vi "Video Write.vi"() -> ()   [LabVIEW 2020, in "examples.lvlib"]
uses:
  examples.lvlib
  common/Image Size (Integer).ctl
  video_io/FourCC.ctl
  video_io/Writer (ARGB)/Writer (ARGB).lvclass/Writer (ARGB).ctl
  common/Image Point (Integer).ctl
  image/Text Drawing Settings.ctl
  image/Font Face.ctl
  image/ARGB Colour.ctl
  video_io/Reader/Reader.lvclass/Reader.ctl
  image/New Image (ARGB Preallocated).vi
  image/Draw Rectangle (ARGB).vi
  image/Draw Text (ARGB).vi
  image/Draw Image to Picture (ARGB).vi
  video_io/Reader/Read Frame (ARGB Next).vi
  video_io/CreateWriter.vi
  image/New Image (ARGB Preallocated).vi/3321fa97-f432-4e1e-8db9-a0df79aed21b.vi
  image/ARGB Colour to U32 Pixel Value.vi
  image/Draw Rectangle (ARGB).vi/7e6fb015-3761-4366-a0a7-e436eb229083.vi
  image/Draw Text (ARGB).vi/0015c4fc-6a12-4f82-815b-6c2f827f408b.vi
  video_io/Writer (ARGB)/Write Frame.vi/0e3f49b0-4303-46d3-b8ab-944fedc4b55e.vi
  image/Draw Image to Picture (ARGB).vi/8cd07b1b-062e-4fe4-9e87-2eb3dc89fe0e.vi
  video_io/Reader/Read Frame (ARGB Next).vi/9eeb12df-7581-4bcd-a397-18dbd97d2298.vi
  <vilib>/Utility/error.llb/Error Cluster From Error Code.vi
  video_io/Writer (ARGB)/Writer (ARGB).lvclass
  video_io/Reader/Reader.lvclass
  video_io/video_io.lvlib
  image/image.lvlib
  common/common.lvlib
panel:
  out "Size":i64 format="%d kB"
  out "Results":cluster{"Input":picture, "Output":picture}[](array[cluster])
  in  "File and Encoding Option":T1(ring)
  # "Different Containers support different encoding types\n(these are just some examples)"
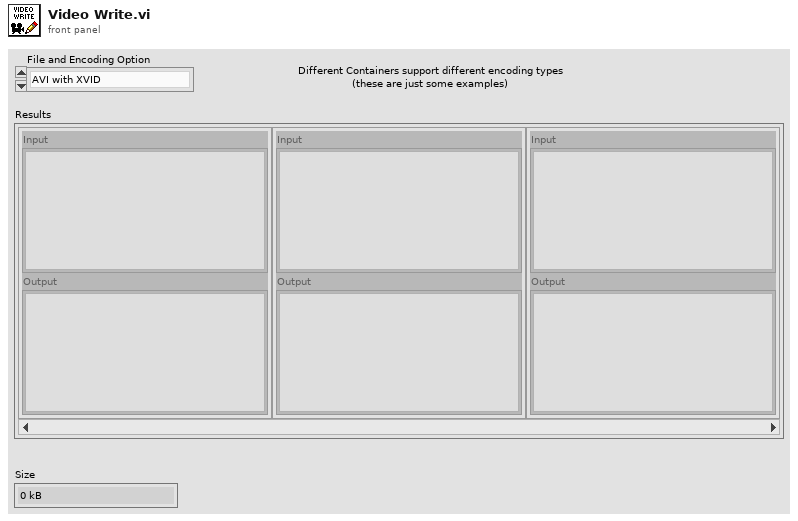
[diagram p1: front panel]
types:
  T1 = enum16{"AVI with XVID", "MKV with RGBA", "MP4 with MP4V"}
  T2 = typedef "common.lvlib/Image Size (Integer).ctl" = cluster{"Width":u16, "Height":u16}
  T3 = typedef "video_io.lvlib/FourCC.ctl" = enum16{"YUV2", "2VUY", "YUVS", "RGBA", "YUV4", "JPEG", "MJPA", "AVDJ", "DMB1", "MP4V", "DIVX", "XVID", "3IV2", "S263", "AVC1", "AI5P", "AI5Q", "AI52", "AI53", "AI55", "AI56", "AI1P", "AI1Q", "AI12", "AI13", "AI15", "AI16", "M1V1", "MPEG", "M2V1", "HDV1", "HDV2", "HDV3", "HDV4", "HDV5", "HDV6", "HDV7", "HDV8", "HDV9", "HDVA", "MX5N", "MX5P", "MX4N", "MX4P", "MX3N", "MX3P", "XD54", "XD55", "XD59", "XD5A", "XD5B", "XD5C", "XD5D", "XD5E", "XD5F", "XDV1", "XDV2", "XDV3", "XDV4", "XDV5", "XDV6", "XDV7", "XDV8", "XDV9", "XDVA", "XDVB", "XDVC", "XDVD", "XDVE", "XDVF", "XDHD", "XDH2", "AVMP", "MJP2", "TIFF", "DRAC", "3IVD", "L555", "L565", "B565", "24BG", "BGRA", "ABGR", "B16G", "B48R", "BXBG", "BXRG", "BXYV", "NO16", "DVOO", "R420", "R411", "WRAW", "AV1X", "AVUP"}
  T4 = typedef "image.lvlib/ARGB Image.ctl" = refnum<data-value>
  T5 = typedef "common.lvlib/Image Point (Integer).ctl" = cluster{"x":i32, "y":i32}
  T6 = typedef "image.lvlib/ARGB Colour.ctl" = cluster{"Alpha":u8, "RGB":u32}
  T7 = typedef "image.lvlib/Text Drawing Settings.ctl" = cluster{"OpenCV Font Face":T8, "Font Scale":dbl}
  T8 = typedef "image.lvlib/Font Face.ctl" = enum8{"FONT_HERSHEY_SIMPLEX", "FONT_HERSHEY_PLAIN", "FONT_HERSHEY_DUPLEX", "FONT_HERSHEY_COMPLEX", "FONT_HERSHEY_TRIPLEX", "FONT_HERSHEY_COMPLEX_SMALL", "FONT_HERSHEY_SCRIPT_SIMPLEX", "FONT_HERSHEY_SCRIPT_COMPLEX", "FONT_ITALIC"}
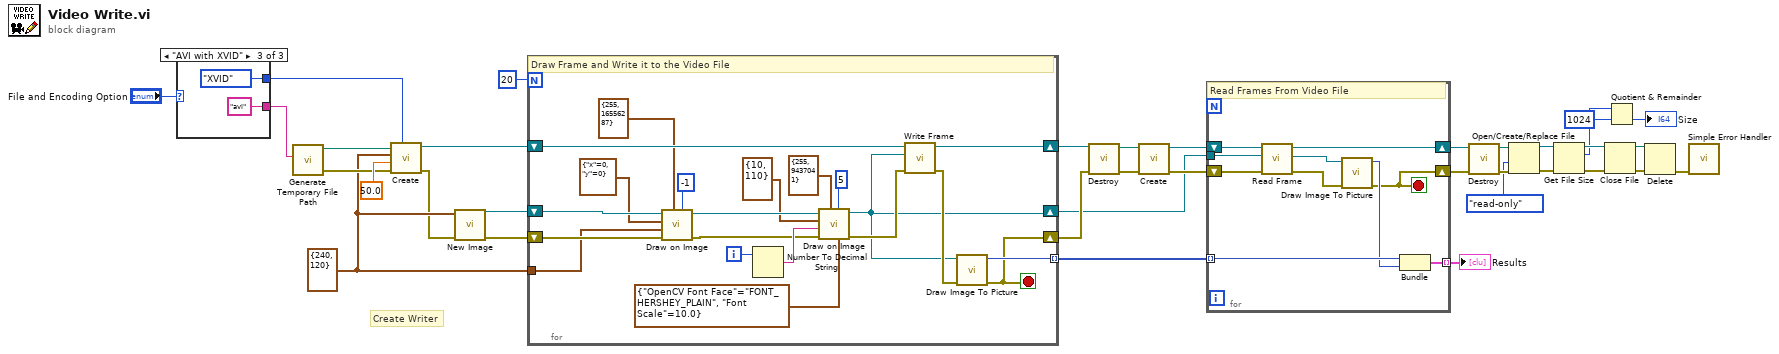
[diagram p0: block diagram]
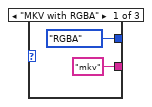
[diagram p2: hidden frame]
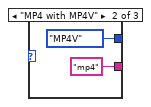
[diagram p3: hidden frame]
diagram:
  w21 = T2 {"Width"=240, "Height"=120} ("Preallocated Image Size (Default: 0,0)")
  # "Create Writer"
  n1 = case shown="\"AVI with XVID\"" "File and Encoding Option" {
    tunnel: ["mkv" "mp4" "avi"] -> w32
    tunnel: [FourCC."RGBA" ("Fourcc") FourCC."MP4V" ("Fourcc") FourCC."XVID" ("Fourcc")] -> w31
    frame "MKV with RGBA" {
    }
    frame "MP4 with MP4V" {
    }
    frame "AVI with XVID" {
    }
  }
  n2 = call <vilib>:"Generate Temporary File Path.vi"("Temporary File Extension (tmp)"=w32) -> ("error out"=w22:errorcluster, "Unique Temporary File Path"=w20:path)  [unwired: 9 in]
  n3 = call "Create.vi"("Fourcc"=w31, "error in (no error)"=w22, "Frames Per Second"=50.0, "Image Size"=w21, "Path"=w20) -> ("error out"=w18:errorcluster, "Writer (ARGB)"=w36:refnum<class "Writer (ARGB).lvclass">)  [unwired: 5 in]
  n4 = call-poly "New Image.vi"("error in (no error)"=w18, "Preallocated Image Size (Default: 0,0)"=w21) -> ("error out"=w17:errorcluster, "ARGB Image"=w27:T4)  [unwired: 8 in]
  n5 = for {
    N: 20 -> [_]
    shift-right: [w53] -> w24
    shift-left: w36 -> [w51]
    shift-right: [w43] -> w34
    shift-left: w17 -> [w55]
    tunnel: w21 -> [w48]
    tunnel: [w45] -> w15 mode=indexing
    shift-right: [w44] -> w16
    shift-left: w27 -> [w61]
    i -> [w57]
    stop <- w43 stop-if-true
    # "Draw Frame and Write it to the Video File"
    n6 = call-poly "Draw on Image.vi"("Thickness (Default: 1)"=-1, "ARGB Colour"=T6 {"Alpha"=255, "RGB"=16556287}, "error in (no error)"=w55, "Point B"=w48, "Point A"=T5 {"x"=0, "y"=0}, "ARGB Image in"=w61) -> ("error out"=w54:errorcluster, "ARGB Image"=w60:T4)  [unwired: 4 in]
    n7 = Number To Decimal String(number=w57) -> (decimal integer string=w56:string)  [unwired: 1 in]
    n8 = call-poly "Draw on Image.vi"("Text Drawing Settings (Default: Simplex)"=T7 {"OpenCV Font Face"=enum."FONT_HERSHEY_PLAIN", "Font Scale"=10.0}, "Thickness (Default: 1)"=5, "ARGB Colour"=T6 {"Alpha"=255, "RGB"=9437041}, "error in (no error)"=w54, "Text"=w56, "Origin"=T5 {"x"=10, "y"=110}, "ARGB Image in"=w60) -> ("error out"=w62:errorcluster, "ARGB Image"=w44:T4)  [unwired: 3 in]
    n9 = call "Write Frame.vi"("error in (no error)"=w62, "ARGB Image in"=w44, "Writer (ARGB) in"=w51) -> ("error out"=w63:errorcluster, "Writer (ARGB)"=w53:refnum<class "Writer (ARGB).lvclass">)  [unwired: 7 in]
    n10 = call-poly "Draw Image To Picture.vi"("error in (no error)"=w63, "ARGB Image Source in"=w44) -> ("error out"=w43:errorcluster, "Picture"=w45:picture)  [unwired: 8 in]
  }
  n11 = call "Destroy.vi"("error in (no error)"=w34, "Writer (ARGB) in"=w24) -> ("error out"=w30:errorcluster, "Path"=w19:path)  [unwired: 8 in]
  n12 = call "Create.vi"("error in (no error)"=w30, "Path"=w19) -> ("error out"=w29:errorcluster, "Reader"=w28:refnum<class "Reader.lvclass">)  [unwired: 8 in]
  n13 = for {
    shift-right: [w64] -> w25
    shift-left: w29 -> [w73]
    shift-right: [w69] -> w26
    shift-left: w28 -> [w72]
    tunnel: w16 -> [w68]
    tunnel: w15 -> [w67] mode=indexing
    tunnel: [w65] -> w13 mode=indexing
    stop <- w64 stop-if-true
    # "Read Frames From Video File"
    n14 = call-poly "Read Frame.vi"("error in (no error)"=w73, "ARGB Image in"=w68, "Reader in"=w72) -> ("error out"=w71:errorcluster, "ARGB Image"=w70:T4, "Reader"=w69:refnum<class "Reader.lvclass">)  [unwired: 6 in]
    n15 = call-poly "Draw Image To Picture.vi"("error in (no error)"=w71, "ARGB Image Source in"=w70) -> ("error out"=w64:errorcluster, "Picture"=w66:picture)  [unwired: 8 in]
    n16 = Bundle("Picture"=w67, "Picture"=w66) -> (w65:cluster{"Picture":picture, "Picture":picture})  [unwired: 1 in]
  }
  "Results" <- w13
  n17 = call "Destroy.vi"("error in (no error)"=w25, "Reader in"=w26) -> ("error out"=w11:errorcluster, "Path"=w10:path)  [unwired: 8 in]
  n18 = Open/Create/Replace File(file path (use dialog)=w10, error in=w11, access (0:read/write)=enum16{"read/write", "read-only", "write-only"}."read-only") -> (refnum out=w8:refnum<file>, error out=w7:errorcluster)  [unwired: 3 in, 1 out]
  n19 = Get File Size(file=w8, error in=w7) -> (refnum out=w12:refnum<file>, size (in bytes)=w3:i64, 0:w5:errorcluster)
  n20 = Close File(refnum=w12, error in=w5) -> (path=w6:path, error out=w4:errorcluster)
  n21 = Quotient & Remainder(x=w3, y=i64 1024) -> (floor(x/y)=→"Size":i64)  [unwired: 1 out]
  n22 = Delete(path (use dialog)=w6, error in=w4) -> (error out=w14:errorcluster)  [unwired: 3 in, 2 out]
  n23 = call <vilib>:"Simple Error Handler.vi"("error in (no error)"=w14) -> ()  [unwired: 4 in, 5 out]
